vi "Read AD Data.vi"() -> ()   [LabVIEW 2012]
uses:
  demo dll.dll
panel:
  out "SampleRate":dbl
  out "Wave":dbl[](graph)=[6.1009628528477355, 0.5814646800632639, 4.268965284839781, 1.0372794052051892, 6.6105216837639125, 6.156450655214087, 8.593245142711767, 5.01006843435418, 3.0487945035421826, 0.2517464427280247, 5.368993661633943, 5.061790484007798, 0.12003027424143387, 4.2586087367964955, 0.26222331936988086, 7.017371700016344, 1.185992291202873, 7.619558737673568, 0.4128132454201694, 7.737314711901693, 4.909649798727818, 8.668819968303193, 5.857096676877758, 3.8449667777872554, 2.8275826347035604, 0.04246640501212262, 8.268991693494648, 3.031581480432979, 6.435679543127061, 4.3401200584622925, 4.4661319060834614, 2.2567164211280177, 3.569572382883288, 5.688431781654022, 0.5112296305222586, 6.345361964197336, 5.530580325427987, 7.94728014322323, 7.022871524746144, 4.274721321510335, 1.203466032363616, 8.812900776784737, 8.167212018687739, 2.798283841978688, 7.746862367509917, 9.867127917017694, 2.717265837023115, 1.4742820520734967, 6.583142514453484, 8.057686972118038, 6.397413373791975, 1.3544606136324466, 8.110388077509265, 7.400629523791245, 4.306597210651062, 6.0643524607183386, 1.3364367944649769, 6.782660159714846, 9.473867993616045, 9.009546878574872, 7.354393341477001, 6.255301795983845, 1.6518697944400262, 0.7081759178541214, 7.1641290470848284, 7.637327070316228, 4.136826022028785, 2.3870730383714345, 4.7608282267525865, 9.066993114129072, 2.668539062827451, 5.757473604092107, 2.250659465498621, 9.544507401111517, 2.3020689964933183, 5.037026616384061, 0.683997448140572, 9.90707490473193, 5.268265305400597, 8.79590955975102, 0.33913964037284305, 6.457850225313706, 2.504770291633922, 1.1771444730299274, 9.856169486143479, 6.396464537339739, 7.937572735207152, 2.9901654822576806, 2.7446947421756107, 5.910913295757709, 9.204255282457794, 8.145497183602611, 5.873487799224417, 8.377801279512623, 5.453233215037829, 3.9604319617695083, 4.687121124480802, 1.6851042636077773, 9.045331534829451, 2.6461141592306836, 1.6058748105761023, 0.8749104331018298, 4.919638614332404, 3.1694695291353536, 2.561268457423438, 1.581890435492641, 6.342629245332052, 1.9138760606674432, 9.148840731034547, 4.251331222180543, 3.1846888054026268, 8.076687021153123, 2.233205926704789, 3.9103361596102792, 2.8853939449649735, 6.660261447960822, 1.3979803671938007, 0.8497730144209248, 5.950047452926053, 6.341156009519021, 2.013392502534632, 9.249415148710597, 9.826699428705568, 6.949504989712352, 3.08893374471211, 0.35780847848670305, 9.038557175877738, 1.3853917536395333, 7.098159920876541, 9.442302363453086, 3.300401126928836, 8.988630818227994, 2.889313262209028, 9.195756171100411, 4.72130097659182, 3.788135340961558, 0.03491022423093737, 8.835563364711764, 8.479537536431137, 9.230840594691013, 3.675547659862186, 4.6209591616104495, 6.367310332648579, 1.9718431753230026, 9.004967057272594, 1.8767308969417518, 3.793094094885918, 0.7545744166465407, 8.850428791142463, 9.691186167555738, 6.5302967239906895, 7.78209303857242, 0.0097322716827275, 9.058948124969731, 9.982635199206308, 3.7921431044512177, 1.627241459935409, 5.698899782438936, 5.868220194210942, 3.899579960957542, 5.340829365217896, 6.591991721283808, 9.24616352459173, 1.0433777406145683, 5.582164582060612, 3.9377680331446685, 1.8717159449173315, 7.499762564634991, 4.388520281128652, 1.732433760589891, 1.7760955522803457, 5.529126354284921, 1.8880824868262103, 1.369488966210115, 9.112409071873707, 8.31219051315755, 5.015739563373629, 0.9539322108944592, 3.714654196678817, 3.2226494885303425, 5.535507287318726, 2.0263674877884985, 0.10489431508585056, 4.658904974064479, 6.97278573556932, 4.348149323703467, 5.1168288020241555, 4.167477540257069, 0.004297272718398748, 1.422987331647898, 7.427530683639139, 9.564016786743467, 2.0717141656071414, 8.628223278907878, 7.862895496733097, 2.359519797598175, 3.0383622894401574, 8.883654935601765, 9.467010466391203, 7.57980075064131, 3.369858556483849, 4.4683663891211856, 8.484902318586053, 6.2952644447831485, 7.549730655229486, 0.8132238723023733, 3.745801968180395, 9.237257204762896, 1.3631600815251477, 8.297586313445589, 3.0472099149717558, 7.28612730228302, 3.9058253972403945, 1.4924732951599862, 6.779810887602728, 8.519805180967632, 8.264107290031166, 0.7674040824274941, 6.355643561574165, 9.238675812014229, 0.7844839138478354, 9.354279571699102, 0.8546333523869287, 3.2629169188773055, 5.75911967260426, 5.777703027681702, 7.5767962816195755, 3.9593063837942477, 5.647288277724827, 3.264236413570336, 3.4222081617665068, 7.526271008926198, 0.6699693223851222, 1.8459763573934573, 2.0324444209608394, 3.31666317680817, 6.984735749805429, 2.244824718746423, 5.1562042106413495, 2.7572393209350787, 5.304726624509488, 8.078422479884523, 9.896025191451, 6.595755203845242, 0.03689692451457116, 7.888393226700078, 9.923147386641126, 1.0424265982913883, 8.099023442951443, 4.912072011763257, 2.0470003198669917, 4.505843129588003, 1.077162858059535, 4.49288021898377, 9.84898283715448, 5.466437756922653, 0.0, 0.0, 0.0, 0.0, 0.0, 0.0, 0.0, 0.0, 0.0, 0.0, 0.0, 0.0, 0.0, 0.0, 0.0, 0.0, 0.0, 0.0, 0.0, 0.0, 0.0, 0.0, 0.0, 0.0, 0.0, 0.0, 0.0, 0.0, 0.0, 0.0, 0.0, 0.0, 0.0, 0.0, 0.0, 0.0, 0.0, 0.0, 0.0, 0.0, 0.0, 0.0]
  in  "Scale":dbl=10.0
  out "ADData":dbl[](array[numeric])=[1000.0, 10.0, 6.1009628528477355, 0.5814646800632639, 4.268965284839781, 1.0372794052051892, 6.6105216837639125, 6.156450655214087, 8.593245142711767, 5.01006843435418, 3.0487945035421826, 0.2517464427280247, 5.368993661633943, 5.061790484007798, 0.12003027424143387, 4.2586087367964955, 0.26222331936988086, 7.017371700016344, 1.185992291202873, 7.619558737673568, 0.4128132454201694, 7.737314711901693, 4.909649798727818, 8.668819968303193, 5.857096676877758, 3.8449667777872554, 2.8275826347035604, 0.04246640501212262, 8.268991693494648, 3.031581480432979, 6.435679543127061, 4.3401200584622925, 4.4661319060834614, 2.2567164211280177, 3.569572382883288, 5.688431781654022, 0.5112296305222586, 6.345361964197336, 5.530580325427987, 7.94728014322323, 7.022871524746144, 4.274721321510335, 1.203466032363616, 8.812900776784737, 8.167212018687739, 2.798283841978688, 7.746862367509917, 9.867127917017694, 2.717265837023115, 1.4742820520734967, 6.583142514453484, 8.057686972118038, 6.397413373791975, 1.3544606136324466, 8.110388077509265, 7.400629523791245, 4.306597210651062, 6.0643524607183386, 1.3364367944649769, 6.782660159714846, 9.473867993616045, 9.009546878574872, 7.354393341477001, 6.255301795983845, 1.6518697944400262, 0.7081759178541214, 7.1641290470848284, 7.637327070316228, 4.136826022028785, 2.3870730383714345, 4.7608282267525865, 9.066993114129072, 2.668539062827451, 5.757473604092107, 2.250659465498621, 9.544507401111517, 2.3020689964933183, 5.037026616384061, 0.683997448140572, 9.90707490473193, 5.268265305400597, 8.79590955975102, 0.33913964037284305, 6.457850225313706, 2.504770291633922, 1.1771444730299274, 9.856169486143479, 6.396464537339739, 7.937572735207152, 2.9901654822576806, 2.7446947421756107, 5.910913295757709, 9.204255282457794, 8.145497183602611, 5.873487799224417, 8.377801279512623, 5.453233215037829, 3.9604319617695083, 4.687121124480802, 1.6851042636077773, 9.045331534829451, 2.6461141592306836, 1.6058748105761023, 0.8749104331018298, 4.919638614332404, 3.1694695291353536, 2.561268457423438, 1.581890435492641, 6.342629245332052, 1.9138760606674432, 9.148840731034547, 4.251331222180543, 3.1846888054026268, 8.076687021153123, 2.233205926704789, 3.9103361596102792, 2.8853939449649735, 6.660261447960822, 1.3979803671938007, 0.8497730144209248, 5.950047452926053, 6.341156009519021, 2.013392502534632, 9.249415148710597, 9.826699428705568, 6.949504989712352, 3.08893374471211, 0.35780847848670305, 9.038557175877738, 1.3853917536395333, 7.098159920876541, 9.442302363453086, 3.300401126928836, 8.988630818227994, 2.889313262209028, 9.195756171100411, 4.72130097659182, 3.788135340961558, 0.03491022423093737, 8.835563364711764, 8.479537536431137, 9.230840594691013, 3.675547659862186, 4.6209591616104495, 6.367310332648579, 1.9718431753230026, 9.004967057272594, 1.8767308969417518, 3.793094094885918, 0.7545744166465407, 8.850428791142463, 9.691186167555738, 6.5302967239906895, 7.78209303857242, 0.0097322716827275, 9.058948124969731, 9.982635199206308, 3.7921431044512177, 1.627241459935409, 5.698899782438936, 5.868220194210942, 3.899579960957542, 5.340829365217896, 6.591991721283808, 9.24616352459173, 1.0433777406145683, 5.582164582060612, 3.9377680331446685, 1.8717159449173315, 7.499762564634991, 4.388520281128652, 1.732433760589891, 1.7760955522803457, 5.529126354284921, 1.8880824868262103, 1.369488966210115, 9.112409071873707, 8.31219051315755, 5.015739563373629, 0.9539322108944592, 3.714654196678817, 3.2226494885303425, 5.535507287318726, 2.0263674877884985, 0.10489431508585056, 4.658904974064479, 6.97278573556932, 4.348149323703467, 5.1168288020241555, 4.167477540257069, 0.004297272718398748, 1.422987331647898, 7.427530683639139, 9.564016786743467, 2.0717141656071414, 8.628223278907878, 7.862895496733097, 2.359519797598175, 3.0383622894401574, 8.883654935601765, 9.467010466391203, 7.57980075064131, 3.369858556483849, 4.4683663891211856, 8.484902318586053, 6.2952644447831485, 7.549730655229486, 0.8132238723023733, 3.745801968180395, 9.237257204762896, 1.3631600815251477, 8.297586313445589, 3.0472099149717558, 7.28612730228302, 3.9058253972403945, 1.4924732951599862, 6.779810887602728, 8.519805180967632, 8.264107290031166, 0.7674040824274941, 6.355643561574165, 9.238675812014229, 0.7844839138478354, 9.354279571699102, 0.8546333523869287, 3.2629169188773055, 5.75911967260426, 5.777703027681702, 7.5767962816195755, 3.9593063837942477, 5.647288277724827, 3.264236413570336, 3.4222081617665068, 7.526271008926198, 0.6699693223851222, 1.8459763573934573, 2.0324444209608394, 3.31666317680817, 6.984735749805429, 2.244824718746423, 5.1562042106413495, 2.7572393209350787, 5.304726624509488, 8.078422479884523, 9.896025191451, 6.595755203845242, 0.03689692451457116, 7.888393226700078, 9.923147386641126, 1.0424265982913883, 8.099023442951443, 4.912072011763257, 2.0470003198669917, 4.505843129588003, 1.077162858059535, 4.49288021898377, 9.84898283715448, 5.466437756922653, 0.0, 0.0, 0.0, 0.0, 0.0, 0.0, 0.0, 0.0, 0.0, 0.0, 0.0, 0.0, 0.0, 0.0, 0.0, 0.0, 0.0, 0.0, 0.0, 0.0, 0.0, 0.0, 0.0, 0.0, 0.0, 0.0, 0.0, 0.0, 0.0, 0.0, 0.0, 0.0, 0.0, 0.0, 0.0, 0.0, 0.0, 0.0, 0.0, 0.0, 0.0, 0.0]
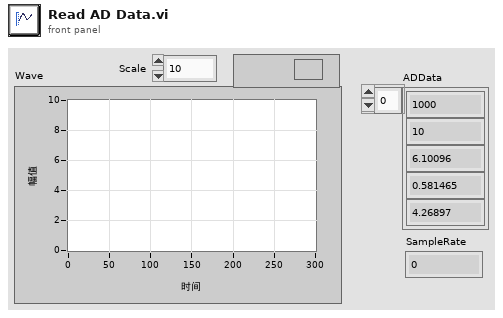
[diagram p1: front panel]
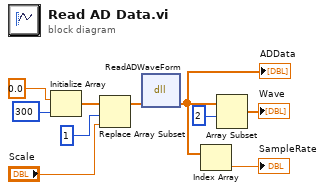
[diagram p0: block diagram]
diagram:
  n1 = Initialize Array(0.0 ("元素"), 300 ("维数大小")) -> (w6:dbl[])
  n2 = Replace Array Subset(array=w6, new element="Scale", index=1) -> (w3:dbl[])
  n3 = dll-call lib="PTH1+abs EBOOK\t功能块DLLdemo dll.dll" fn="ReadADWaveForm"("ADData"=w3) -> ("ADData"=w2:dbl[])  [unwired: 4 in, 2 out]
  "ADData" <- w2
  n4 = Index Array(array=w2) -> (element=→"SampleRate":dbl)  [unwired: 1 in]
  n5 = Array Subset(array=w2, index=2 ("索引")) -> (→"Wave":dbl[])  [unwired: 1 in]
